vi "Launch all modules - Top Level VI.vi"(8 "error in":errorcluster) -> (0 "error out":errorcluster)   [LabVIEW 2018]
uses:
  modules/Common/Common.lvlib
  modules/Common/vi/Stop All - Action.ctl
  modules/Controller/Controller.lvlib
  modules/Error Handler/Error Handler/Error Handler.lvlib
  modules/Entry Console/Entry Console.lvlib
  modules/Wash Display Console/Wash Display Console.lvlib
  modules/Vehicle Position Interface/Vehicle Position Interface.lvlib
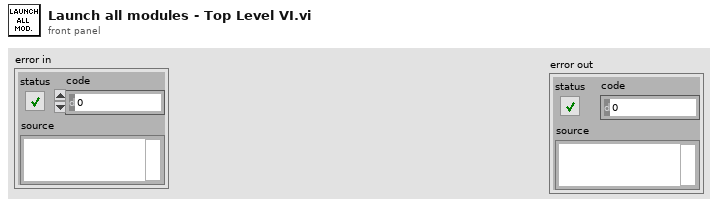
[diagram p1: front panel]
types:
  T1 = typedef "Common.lvlib/Stop All - Action.ctl" = enum16{"Create", "Get", "Fire", "Destroy"}
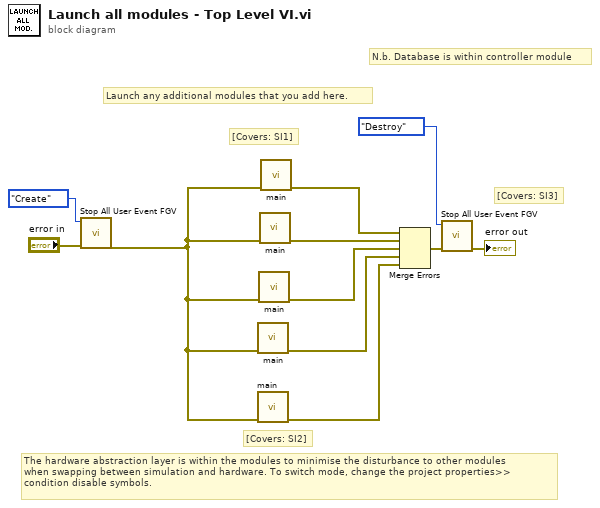
[diagram p0: block diagram]
diagram:
  # "N.b. Database is within controller module"
  # "[Covers: SI1]"
  # "[Covers: SI2]"
  # "[Covers: SI3]"
  # "The hardware abstraction layer is within the modules to minimise the disturbance to other modules\nwhen swapping between simulation and hardware. To switch mode, change the project properties>>\ncondition disable symbols."
  # "Launch any additional modules that you add here."
  n1 = call "Stop All User Event FGV.vi"("error in"="error in", "Action"=Stop_All_-_Action."Create") -> ("error out"=w6:errorcluster)  [unwired: 8 in, 1 out]
  n2 = call "main.vi"("error in"=w6) -> ("error out"=w2:errorcluster)  [unwired: 10 in]
  n3 = call "main.vi"("error in"=w6) -> ("error out"=w1:errorcluster)  [unwired: 10 in]
  n4 = call "main.vi"("error in"=w6) -> ("error out"=w3:errorcluster)  [unwired: 10 in]
  n5 = call "main.vi"("error in"=w6) -> ("error out"=w4:errorcluster)  [unwired: 10 in]
  n6 = call "main.vi"("error in"=w6) -> ("error out"=w5:errorcluster)  [unwired: 10 in]
  n7 = Merge Errors(w5, w4, w3, w2, w1) -> (w7:errorcluster)
  n8 = call "Stop All User Event FGV.vi"("error in"=w7, "Action"=Stop_All_-_Action."Destroy") -> ("error out"=→"error out":errorcluster)  [unwired: 8 in, 1 out]
